vi "UEGO channel.vi"(8 "error in (no error)":errorcluster, 11 "Node Ptr":T2 format="%.0x") -> (0 "error out":errorcluster)   [LabVIEW 2014, in "SLSC configuration System Explorer.lvlib"]
uses:
  SLSC configuration System Explorer.lvlib
  <vilib>/NI Veristand/Custom Device API/Custom Device Item Ref.ctl
  Shared/UEGO Board/Calibration State.ctl
  Shared/Constants.vi
  <vilib>/NI Veristand/Custom Device API/Get Item Property (U16).vi
  <vilib>/NI Veristand/Custom Device API/Custom Device API.lvlib
  Shared/SLSC configuration Shared.lvlib
panel:
  out "Channel #":u8=1
  in  "Initial Value":T1
  in  "Header":cluster{"Section Name":string}={"Section Name"="Calibration Settings"}
  in  "Description":string
  in  "Name":string
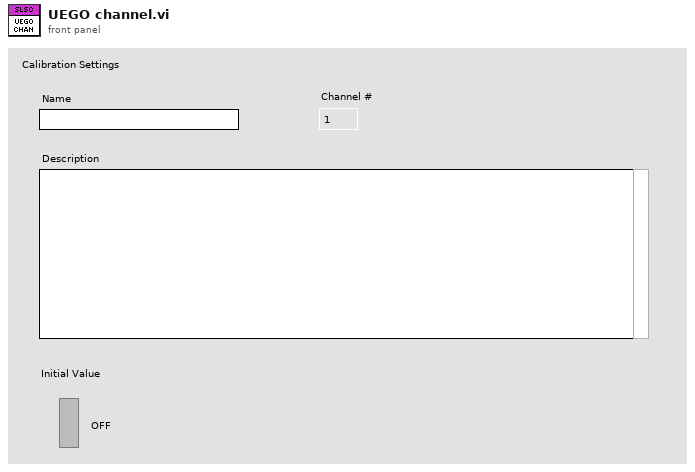
[diagram p1: front panel]
types:
  T1 = typedef "SLSC configuration Shared.lvlib/Calibration State.ctl" = bool
  T2 = typedef "Custom Device API.lvlib/Custom Device Item Ref.ctl" = u64
  T3 = typedef "Custom Device API.lvlib/Custom Device Item Info.ctl" = cluster{"Name":string, "Is Channel":bool, "GUID":string, "Is Waveform":bool}
  T4 = typedef "Custom Device API.lvlib/Custom Device Channel.ctl" = cluster{"Type":T5, "Units":string, "Default Value":dbl, "Faultable":bool, "Scalable":bool}
  T5 = typedef "Custom Device API.lvlib/Custom Device Channel Type.ctl" = enum16{"Input", "Output"}
  T6 = typedef "Custom Device API.lvlib/Custom Device Commands.ctl" = enum16{"Default", "Item renamed", "Shutdown", "Dynamic button pressed"}
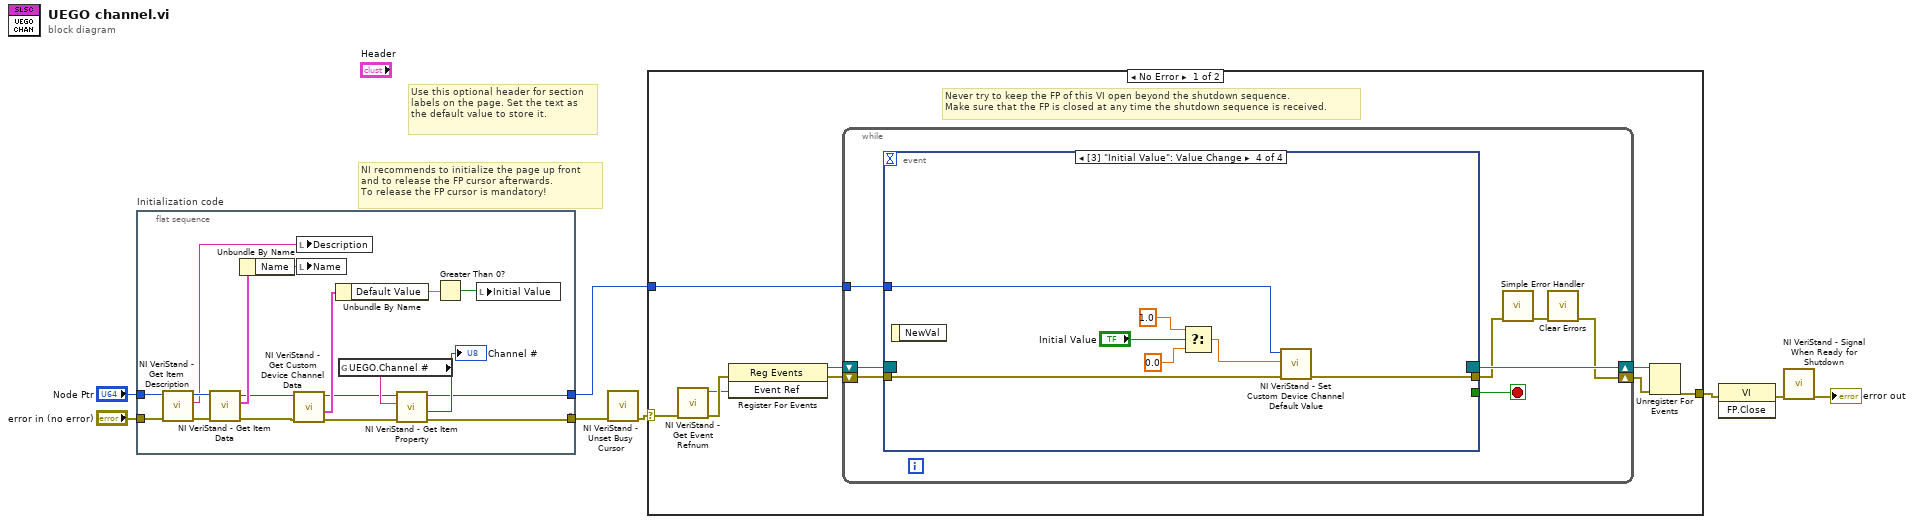
[diagram p0: block diagram]
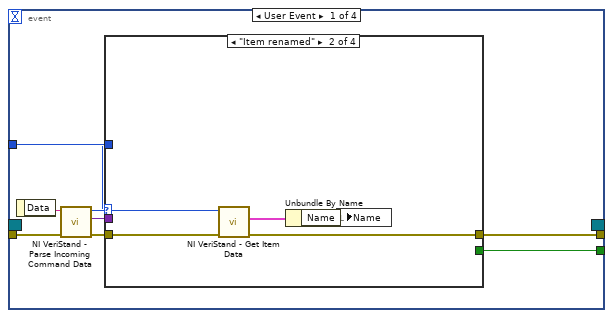
[diagram p2: hidden frame]
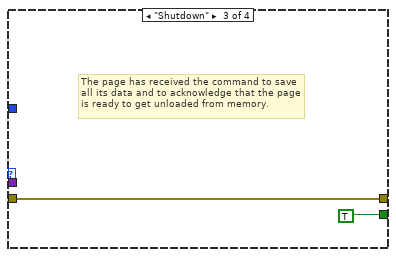
[diagram p4: hidden frame]
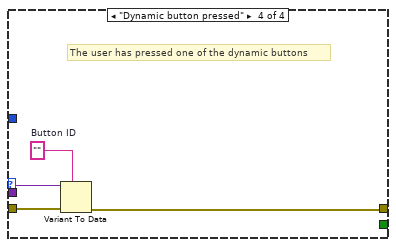
[diagram p5: hidden frame]
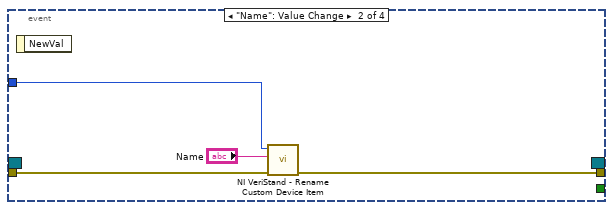
[diagram p6: hidden frame]
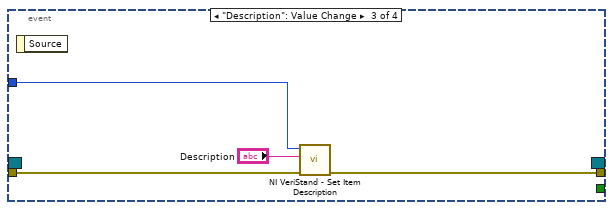
[diagram p7: hidden frame]
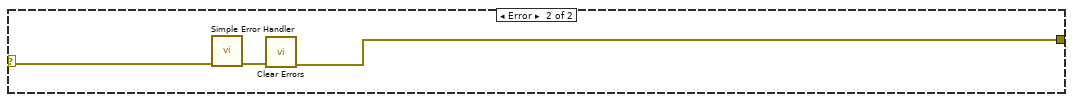
[diagram p8: hidden frame]
diagram:
  # "Use this optional header for section labels on the page. Set the text as the default value to store it."
  # "NI recommends to initialize the page up front\nand to release the FP cursor afterwards.\nTo release the FP cursor is mandatory!"
  n1 = flat-sequence "Initialization code" {
    tunnel: "error in (no error)" -> [w25]
    tunnel: "Node Ptr" -> [w24]
    tunnel: [w12] -> w4
    tunnel: [w11] -> w1
    frame #0 {
      n2 = call <vilib>:"NI VeriStand - Get Item Description.vi"("error in (no error)"=w25, "Item Ref in"=w24) -> ("error out"=w22:errorcluster, "Description"=w23:string, "Item Ref out"=w26:T2)  [unwired: 7 out]
      n3 = call <vilib>:"NI VeriStand - Get Item Data.vi"("error in (no error)"=w22, "Item Ref in"=w26) -> ("error out"=w17:errorcluster, "Item Info"=w21:T3, "Item Ref out"=w18:T2)  [unwired: 7 out]
      n4 = Unbundle By Name(w21) -> ("Name"=w20:string)
      n5 = call <vilib>:"NI VeriStand - Get Custom Device Channel Data.vi"("error in (no error)"=w17, "Channel Ref in"=w18) -> ("error out"=w16:errorcluster, "Channel"=w19:T4, "Channel Ref out"=w13:T2)  [unwired: 4 in, 3 out]
      n6 = local write "Description"(w23) -> ()
      n7 = local write "Name"(w20) -> ()
      n8 = Unbundle By Name(w19) -> ("Default Value"=w10:dbl)
      n9 = global read "Constants.vi" "UEGO.Channel #"() -> (w15:string)
      n10 = call-poly <vilib>:"NI VeriStand - Get Item Property.vi"("error in (no error)"=w16, "Property Name"=w15, "Item Ref in"=w13) -> ("error out"=w12:errorcluster, "Value"=→"Channel #":u16, "Item Ref out"=w11:T2)  [unwired: 5 in, 1 out]
      n11 = Greater Than 0?(x=w10) -> (x > 0?=w9:bool)
      n12 = local write "Initial Value"(w9) -> ()
    }
  }
  n13 = call <vilib>:"NI VeriStand - Unset Busy Cursor.vi"("error in (no error)"=w4) -> ("error out"=w3:errorcluster)  [unwired: 10 out]
  n14 = case shown="No Error" w3 {
    selector: w3 -> [w27 w81]
    tunnel: [w32 w79] -> w8
    tunnel: w1 -> [w28 _]
    frame No Error {
      # "Never try to keep the FP of this VI open beyond the shutdown sequence.\nMake sure that the FP is closed at any time the shutdown sequence is received."
      n15 = call <vilib>:"NI VeriStand - Get Event Refnum.vi"("error in (no error)"=w27) -> ("error out"=w35:errorcluster, "Event Ref"=w31:refnum<user-event>)  [unwired: 9 out]
      n16 = register-events(error in=w35, w31) -> (reference out=w29:refnum<event-registration>, error out=w30:errorcluster)  [unwired: 1 in]
      n17 = while {
        tunnel: w28 -> [w39]
        shift-right: [w36] -> w33
        shift-left: w30 -> [w42]
        shift-right: [w43] -> w34
        shift-left: w29 -> [w41]
        stop <- w40 stop-if-true
        n18 = event shown="[3] \"Initial Value\": Value Change" {
          selector: w41 -> [_ _ _ _]
          dyn-events: [_ _ _ _] -> w43
          timeout: _ -> [_ _ _ _]
          tunnel: w42 -> [w51 w67 w70 w77]
          tunnel: [w47 _ _ _] -> w40
          tunnel: [w46 w66 w69 w76] -> w38
          tunnel: w39 -> [w45 w65 w71 w78]
          event User Event {
            n19 = event-data() -> ("Data"=w50:string)  [unwired: 1 out]
            n20 = call <vilib>:"NI VeriStand - Parse Incoming Command Data.vi"("error in (no error)"=w51, "Incoming data"=w50) -> ("error out"=w49:errorcluster, "Outgoing data"=w44:variant, "Action"=w48:T6)  [unwired: 7 out]
            n21 = case shown="\"Item renamed\"" w48 {
              tunnel: w49 -> [w52 w57 w58 w63]
              tunnel: [_ _ TRUE _] -> w47
              tunnel: [w52 w54 w58 w60] -> w46
              tunnel: w45 -> [_ w56 _ _]
              tunnel: w44 -> [_ _ _ w62]
              frame "Default", Default {
              }
              frame "Item renamed" {
                n22 = call <vilib>:"NI VeriStand - Get Item Data.vi"("error in (no error)"=w57, "Item Ref in"=w56) -> ("error out"=w54:errorcluster, "Item Info"=w55:T3)  [unwired: 8 out]
                n23 = Unbundle By Name(w55) -> ("Name"=w53:string)
                n24 = local write "Name"(w53) -> ()
              }
              frame "Shutdown" {
                # "The page has received the command to save all its data and to acknowledge that the page is ready to get unloaded from memory."
              }
              frame "Dynamic button pressed" {
                w61 = ""  # Button ID
                # "The user has pressed one of the dynamic buttons"
                n25 = Variant To Data(error in=w63, type=w61, Variant=w62) -> (error out=w60:errorcluster)  [unwired: 1 out]
              }
            }
          }
          event "Name": Value Change {
            n26 = event-data() -> ()  [unwired: 2 out]
            n27 = call <vilib>:"NI VeriStand - Rename Custom Device Item.vi"("error in (no error)"=w67, "New Name"="Name", "Item Ref in"=w65) -> ("error out"=w66:errorcluster)  [unwired: 1 in, 7 out]
          }
          event "Description": Value Change {
            n28 = event-data() -> ()  [unwired: 2 out]
            n29 = call <vilib>:"NI VeriStand - Set Item Description.vi"("error in (no error)"=w70, "Description"="Description", "Item Ref in"=w71) -> ("error out"=w69:errorcluster)  [unwired: 8 out]
          }
          event Value Change {
            n30 = event-data() -> ()  [unwired: 2 out]
            n31 = Select(t=1.0, s="Initial Value", f=0.0) -> (s? t:f=w72:dbl)
            n32 = call <vilib>:"NI VeriStand - Set Custom Device Channel Default Value.vi"("error in (no error)"=w77, "Default Value"=w72, "Channel Ref in"=w78) -> ("error out"=w76:errorcluster)  [unwired: 7 in, 1 out]
          }
        }
        n33 = call <vilib>:"Simple Error Handler.vi"("error in (no error)"=w38) -> ("error out"=w37:errorcluster)  [unwired: 1 in, 7 out]
        n34 = call <vilib>:"Clear Errors.vi"("error in (no error)"=w37) -> ("error out"=w36:errorcluster)  [unwired: 1 in, 5 out]
      }
      n35 = Unregister For Events(event registration refnum=w34, error in=w33) -> (error out=w32:errorcluster)
    }
    frame Error {
      n36 = call <vilib>:"Simple Error Handler.vi"("error in (no error)"=w81) -> ("error out"=w80:errorcluster)  [unwired: 1 in, 7 out]
      n37 = call <vilib>:"Clear Errors.vi"("error in (no error)"=w80) -> ("error out"=w79:errorcluster)  [unwired: 1 in, 5 out]
    }
  }
  n38 = invoke class="VI" method="FP.Close"(error in=w8) -> (error out=w7:errorcluster)  [unwired: 2 in, 2 out]
  n39 = call <vilib>:"NI VeriStand - Signal When Ready for Shutdown.vi"("error in (no error)"=w7) -> ("error out"=→"error out":errorcluster)  [unwired: 10 out]
